vi "get&set Homepage.vi"(8 "error in (no error)":errorcluster, 10 "Homepage":string, 11 "VGS_ManufacturerInfo in":refnum<class "VGS_ManufacturerInfo.lvclass">) -> (0 "error out":errorcluster, 2 "Homepage":string, 3 "VGS_ManufacturerInfo out":refnum<class "VGS_ManufacturerInfo.lvclass">)   [LabVIEW 2022 SP3, in "LV_VGS.lvlib" / "VGS_ManufacturerInfo.lvclass"]
uses:
  VGS_ManufacturerInfo.lvclass
  VGS_ManufacturerInfo.lvclass/VGS_ManufacturerInfo.ctl
  C:/Users/Andrey/Desktop/hajo/LV_VGS/vgs_project.dll
  vgs_project.dll
panel:
  in  "Get/Set? (Set)":bool=TRUE
  # "-Set\n-Get"
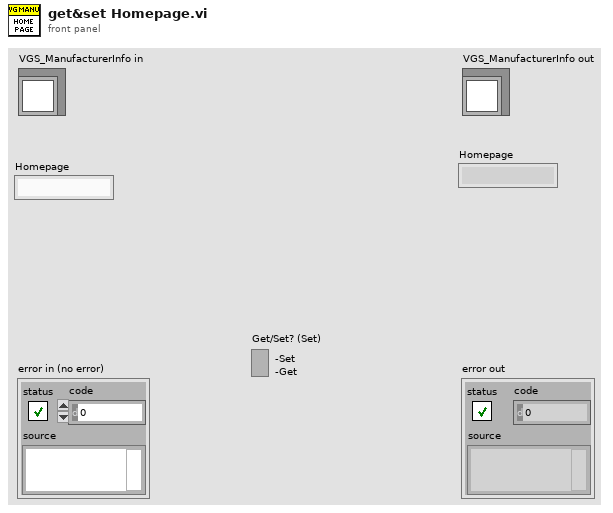
[diagram p1: front panel]
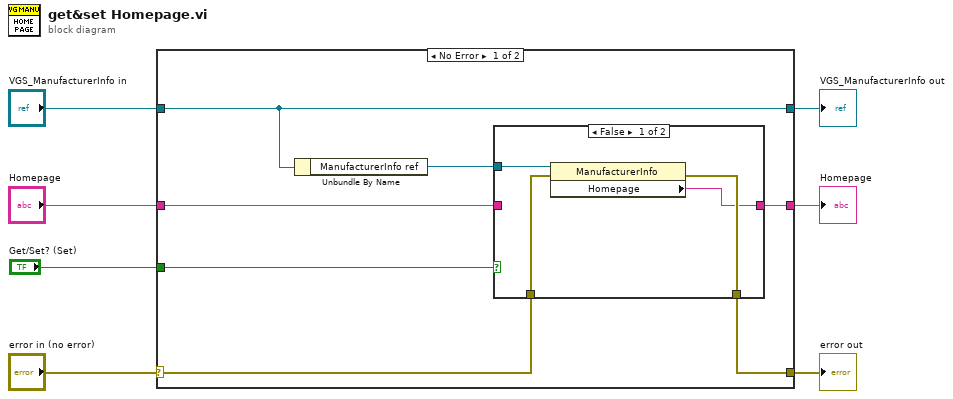
[diagram p0: block diagram]
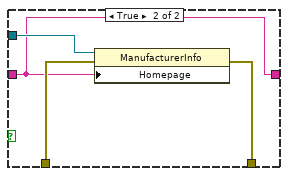
[diagram p2: hidden frame]
diagram:
  n1 = case shown="No Error" "error in (no error)" {
    selector: "error in (no error)" -> [w12 w25]
    tunnel: [w11 w25] -> w4
    tunnel: [w14 w24] -> w5
    tunnel: "VGS_ManufacturerInfo in" -> [w14 w24]
    tunnel: "Get/Set? (Set)" -> [w10 _]
    tunnel: "Homepage" -> [w9 w23]
    tunnel: [w8 w23] -> w1
    frame No Error {
      n2 = Unbundle By Name(w14) -> ("ManufacturerInfo ref"=w13:refnum<k24>)
      n3 = case shown="False" w10 {
        tunnel: w13 -> [w18 w20]
        tunnel: w12 -> [w17 w22]
        tunnel: [w16 w21] -> w11
        tunnel: w9 -> [_ w19]
        tunnel: [w15 w19] -> w8
        frame False {
          n4 = property class="ManufacturerInfo"(reference=w18, error in=w17) -> (error out=w16:errorcluster, "Homepage"=w15:string)  [unwired: 1 out]
        }
        frame True {
          n5 = property class="ManufacturerInfo"(reference=w20, error in=w22, "Homepage"=w19) -> (error out=w21:errorcluster)  [unwired: 1 out]
        }
      }
    }
    frame Error {
    }
  }
  "error out" <- w4
  "VGS_ManufacturerInfo out" <- w5
  "Homepage" <- w1
